vi "code3.vi"() -> ()   [LabVIEW 2019]
panel:
  out "Waveform Chart":dbl(graph)
  in  "B":dbl(knob) scale=0.0..10.0
  in  "A":dbl
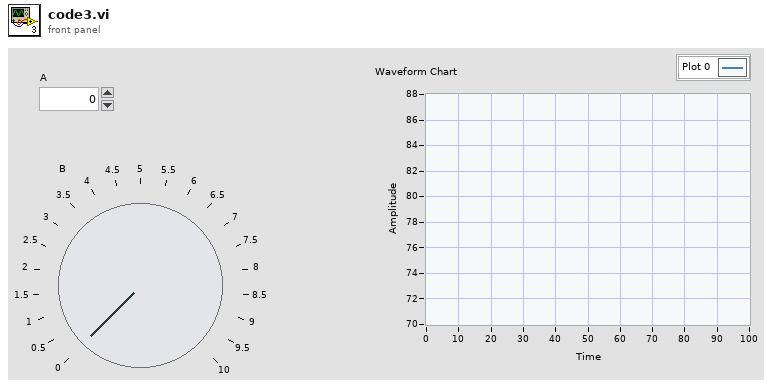
[diagram p1: front panel]
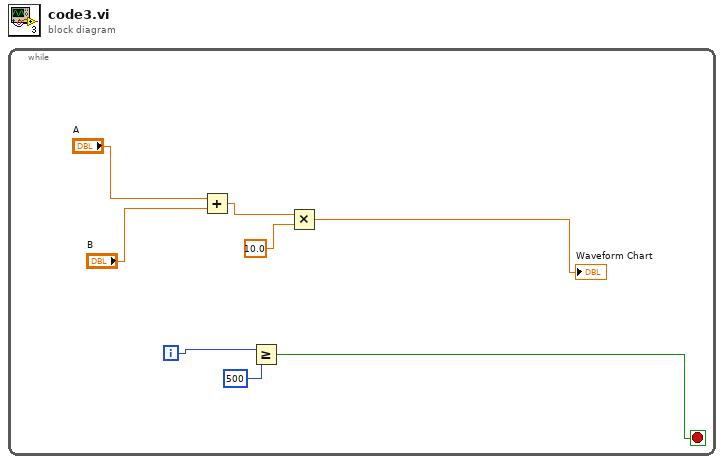
[diagram p0: block diagram]
diagram:
  n1 = while {
    i -> [w3]
    stop <- w1 stop-if-true
    n2 = Add(x="A", y="B") -> (x+y=w6:dbl)
    n3 = Greater Or Equal?(x=w3, y=500) -> (x >= y?=w1:bool)
    n4 = Multiply(x=w6, y=10.0) -> (x*y=→"Waveform Chart":dbl)
  }
